vi "giltch_damaged_detector.vi"(10 "D":ext[](array[numeric]), 11 "side points":dbl[][](array[numeric])) -> (0 "damaged coord":dbl[](array[numeric]), 1 "giltch_coord":dbl[](array[numeric]), 2 "D_damaged":ext, 3 "D_giltch":ext)   [LabVIEW 2017]
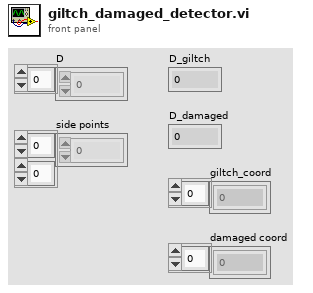
[diagram p1: front panel]
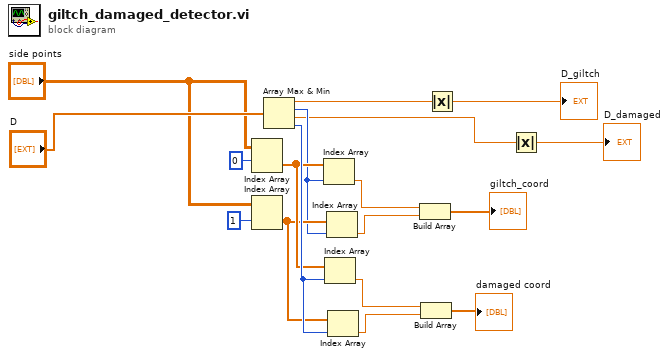
[diagram p0: block diagram]
diagram:
  n1 = Index Array(array="side points", index (row)=0) -> (element=w13:dbl[])  [unwired: 1 in]
  n2 = Index Array(array="side points", index (row)=1) -> (element=w12:dbl[])  [unwired: 1 in]
  n3 = Array Max & Min(array="D") -> (max value=w4:ext, max index (indices)=w7:i32, min value=w2:ext, min index (indices)=w14:i32)
  n4 = Index Array "Index Array"(array=w13, index=w7) -> (element=w8:dbl)
  n5 = Index Array(array=w13, index=w14) -> (element=w11:dbl)
  n6 = Index Array(array=w12, index=w7) -> (element=w9:dbl)
  n7 = Index Array(array=w12, index=w14) -> (element=w10:dbl)
  n8 = Build Array(w8, w9) -> (→"giltch_coord":dbl[])
  n9 = Build Array(w11, w10) -> (→"damaged coord":dbl[])
  n10 = Absolute Value(x=w4) -> (abs(x)=→"D_giltch":ext)
  n11 = Absolute Value(x=w2) -> (abs(x)=→"D_damaged":ext)
